vi "Read Voltage.vi"(8 "error in (no error)":errorcluster, 11 "PS Simulated in":refnum<class "PS Simulated.lvclass">) -> (0 "error out":errorcluster, 2 "Voltage":dbl, 3 "PS Simulated out":refnum<class "PS Simulated.lvclass">)   [LabVIEW 2021, in "PS.lvlib" / "PS Simulated.lvclass"]
uses:
  PS Simulated.lvclass
  PS Simulated.lvclass/PS Simulated.ctl
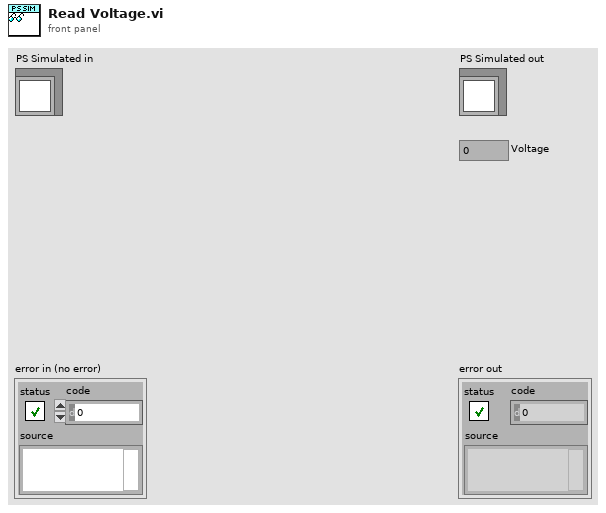
[diagram p1: front panel]
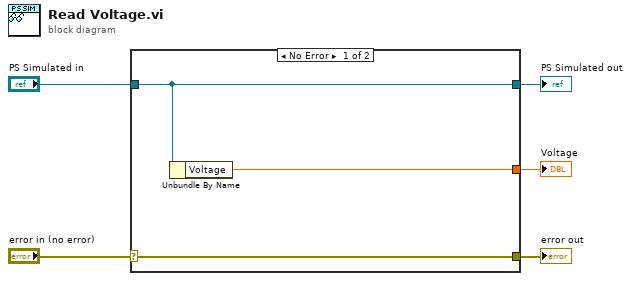
[diagram p0: block diagram]
diagram:
  n1 = case shown="No Error" "error in (no error)" {
    selector: "error in (no error)" -> [w8 w9]
    tunnel: [w8 w9] -> w4
    tunnel: [w7 w10] -> w2
    tunnel: "PS Simulated in" -> [w7 w10]
    tunnel: [w6 _] -> w1
    frame No Error {
      n2 = Unbundle By Name(w7) -> ("Voltage"=w6:dbl)
    }
    frame Error {
    }
  }
  "error out" <- w4
  "PS Simulated out" <- w2
  "Voltage" <- w1
